vi "OP300ZP_CONTI_VI.vi"(6 "Dernier Point en entrée":bool, 7 "OUI/NON":bool, 8 "entrée d'erreur (pas d'erreur)":errorcluster, 9 "Refnum Bool":refnum<vi>, 10 "Refnum NumNb":refnum<vi>, 11 "Cluster en entrée":refnum<vi>) -> (0 "sortie d'erreur":errorcluster, 1 "Dernier Point en sortie":bool, 2 "Compt":i32, 3 "Dernier Point 3":bool)   [LabVIEW 2020]
uses:
  <vilib>/Sylvain.lib/02 SLIM ZEN WS 500/SubVi/FGV.ctl
  VG/R.vi
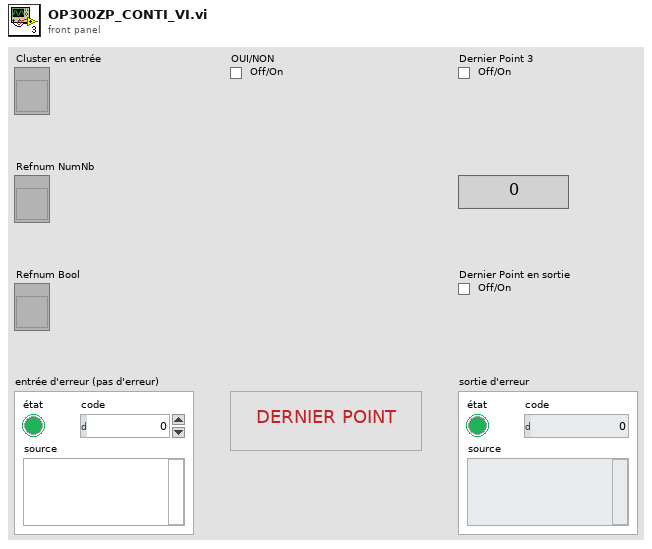
[diagram p1: front panel]
types:
  T1 = typedef "FGV.ctl" = enum16{"GET", "SET", "RAZ"}
  T2 = cluster{"3562":string, "MX5060":string, "ST5520":string}
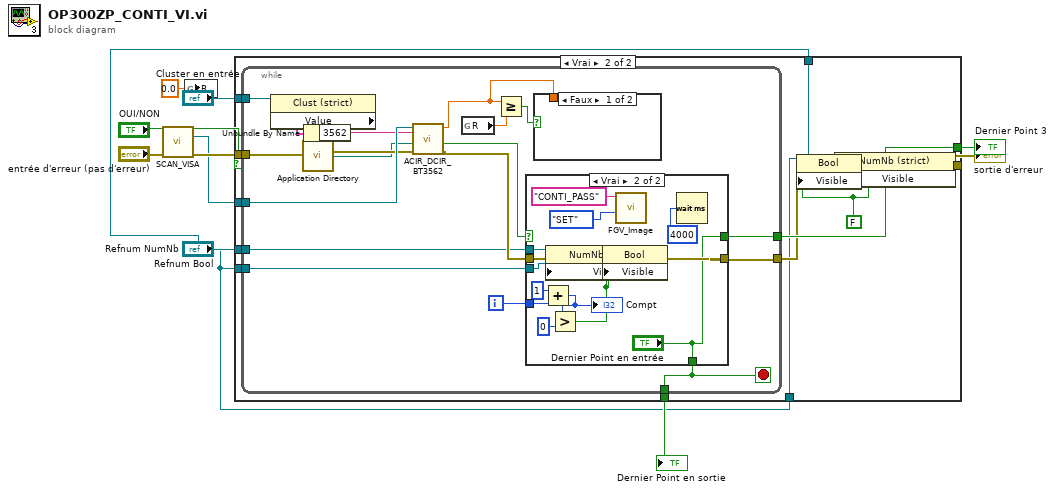
[diagram p0: block diagram]
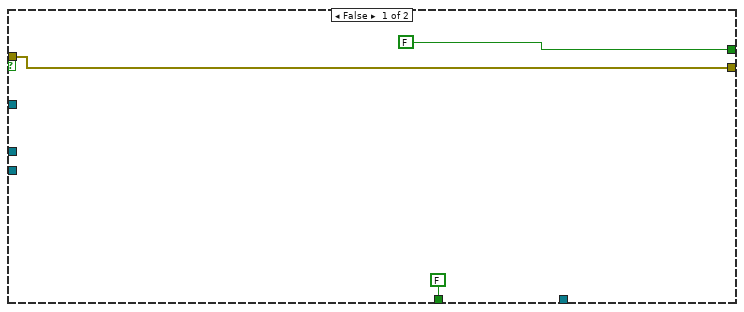
[diagram p2: hidden frame]
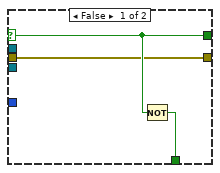
[diagram p3: hidden frame]
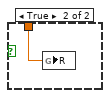
[diagram p4: hidden frame]
diagram:
  n1 = call "SCAN_VISA.vi"("entrée d'erreur (pas d'erreur)"="entrée d'erreur (pas d'erreur)") -> ("sortie d'erreur"=w11:errorcluster, "Refnum VISA en sortie"=w4:refnum<visa-resource-name>)  [unwired: 9 in]
  n2 = global write "R.vi" "R"(0.0 ("R")) -> ()
  n3 = case shown="Vrai" "OUI/NON" {
    tunnel: w4 -> [_ w27]
    tunnel: w11 -> [w14 w26]
    tunnel: [w14 w23] -> w7
    tunnel: [FALSE ("OUI/NON") w25] -> w8
    tunnel: [FALSE w24] -> w10
    tunnel: "Cluster en entrée" -> [_ w19]
    tunnel: "Refnum NumNb" -> [_ w18]
    tunnel: "Refnum Bool" -> [_ w17]
    tunnel: "Refnum NumNb" -> [_ w16]
    tunnel: "Refnum Bool" -> [_ w15]
    frame False {
    }
    frame True {
      w20 = FALSE ("Visible")
      n4 = while {
        tunnel: w27 -> [w44]
        tunnel: w26 -> [w43]
        tunnel: [w40] -> w22
        tunnel: [w35] -> w25
        tunnel: [w34] -> w24
        tunnel: w19 -> [w30]
        tunnel: w18 -> [w29]
        tunnel: w17 -> [w28]
        i -> [w39]
        stop <- w34 stop-if-true
        n5 = property class="Clust (strict)"(reference=w30) -> ("Value"=w32:T2)  [unwired: 1 in, 2 out]
        n6 = call <vilib>:"Application Directory.vi"() -> ("Application Directory"=w42:path)
        n7 = Unbundle By Name(w32) -> ("3562"=w31:string)
        n8 = call <userlib>:"ACIR_DCIR_BT3562.vi"("errin"=w43, "chemin de base"=w42, "section"=w31, "VISAin"=w44) -> ("errout"=w33:errorcluster, "R pass"=w41:bool, "R Out float"=w36:dbl)  [unwired: 5 out]
        n9 = global read "R.vi" "R"() -> (w38:dbl)
        n10 = Greater Or Equal?(x=w36, y=w38) -> (x >= y?=w37:bool)
        n11 = case shown="Vrai" w41 {
          selector: w41 -> [w47 _]
          tunnel: w33 -> [w45 w56]
          tunnel: [w45 w52] -> w40
          tunnel: [w46 "Dernier Point en entrée"] -> w34
          tunnel: w39 -> [_ w59]
          tunnel: [w47 "Dernier Point en entrée"] -> w35
          tunnel: w29 -> [_ w49]
          tunnel: w28 -> [_ w48]
          frame False {
            n12 = Not(x=w47) -> (.not. x?=w46:bool)
          }
          frame True {
            n13 = Add(x=1, y=w59) -> (x+y=w55:i32)
            "Compt" <- w55
            n14 = Greater?(x=w55, y=0) -> (0:w51:bool)
            n15 = property on="Nœud de propriété" class="NumNb (strict)"(reference=w49, error in=w56, "Visible"=w51) -> (error out=w53:errorcluster)  [unwired: 1 out]
            n16 = property on="Nœud de propriété" class="Bool"(reference=w48, error in=w53, "Visible"=w51) -> (error out=w52:errorcluster)  [unwired: 1 out]
            n17 = call <vilib>:"FGV_Image.vi"("Énum"=FGV."SET", "IN"="CONTI_PASS") -> ()  [unwired: 9 in, 1 out]
            n18 = Wait (ms)(milliseconds to wait=u32 4000 ("attente (ms)")) -> ()  [unwired: 1 out]
          }
        }
        n19 = case shown="Faux" w37 {
          tunnel: w36 -> [_ w62]
          frame False {
          }
          frame True {
            n20 = global write "R.vi" "R"(w62) -> ()
          }
        }
      }
      n21 = property on="Nœud de propriété" class="Bool"(reference=w15, error in=w22, "Visible"=w20) -> (error out=w21:errorcluster)  [unwired: 1 out]
      n22 = property on="Nœud de propriété" class="NumNb (strict)"(reference=w16, error in=w21, "Visible"=w20) -> (error out=w23:errorcluster)  [unwired: 1 out]
    }
  }
  "Dernier Point en sortie" <- w10
  "Dernier Point 3" <- w8
  "sortie d'erreur" <- w7
